vi "WPI_CameraRead MJPG for Dashboard.vi"(6 "Camera Settings":T2={"fps"=30, "compression"=30, "Image Size"=enum."320x240"}, 7 "port":u16=1180, 8 "Rec Mode":u16(ring) items=["O", "*", "Open Playback Panel"], 9 "Camera IP":string, 10 "Camera Mode":u16(ring) items=["Camera Off", "USB Camera SW", "USB Camera HW", "IP Camera"], 11 "Refnum in":T1) -> (2 "Active":bool, 3 "Refnum out":T1, 4 "FPS":dbl, 5 "Bandwidth (Mbps)":dbl)   [LabVIEW 2015]
uses:
  <vilib>/Rock Robotics/WPI/Camera/WPI_CameraSettings Read MJPG.ctl
  <vilib>/Rock Robotics/WPI/Camera/WPI_CameraImageSize.ctl
  <vilib>/vision/Image Controls.llb/IMAQ Image.ctl
  <vilib>/Rock Robotics/WPI/Dashboard/WPI_DashboardLogging Global.vi
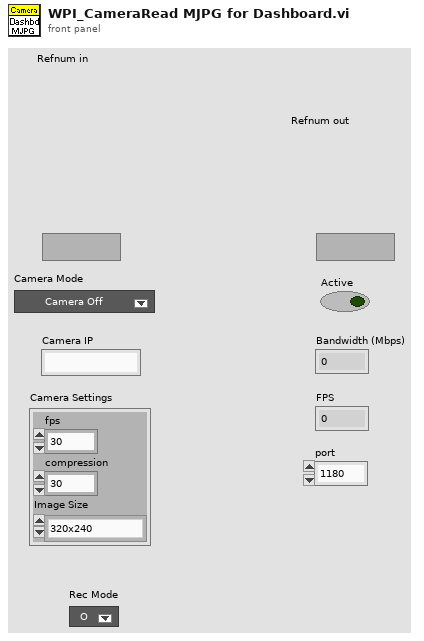
[diagram p1: front panel]
types:
  T1 = typedef "IMAQ Image.ctl" = refnum<image>
  T2 = typedef "WPI_CameraSettings Read MJPG.ctl" = cluster{"fps":i32, "compression":i32, "Image Size":T3}
  T3 = typedef "WPI_CameraImageSize.ctl" = enum16{"640x480", "320x240", "160x120", "Custom"}
  T4 = typedef "IMAQ AVI2 Refnum.ctl" = refnum<k20>
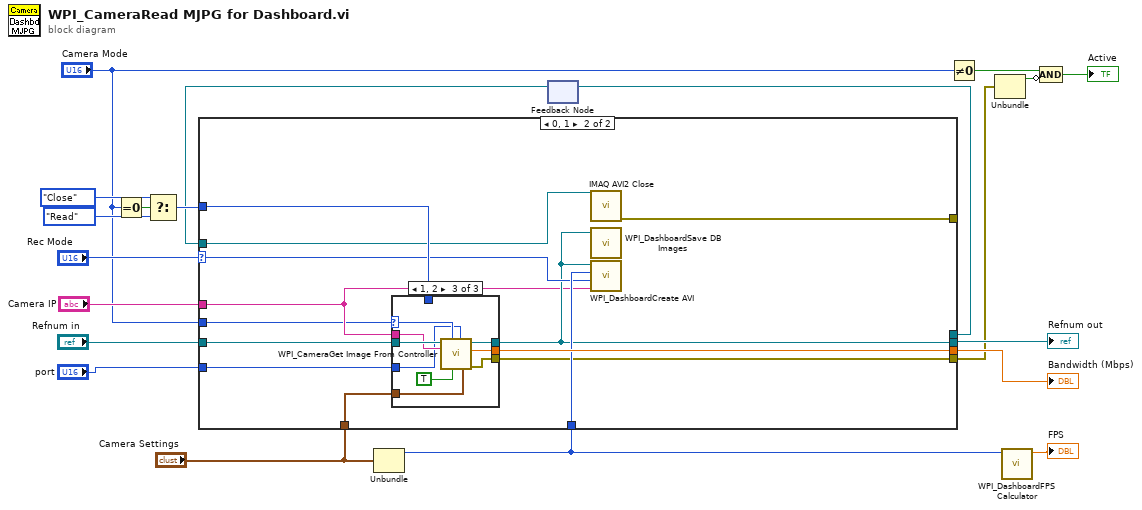
[diagram p0: block diagram]
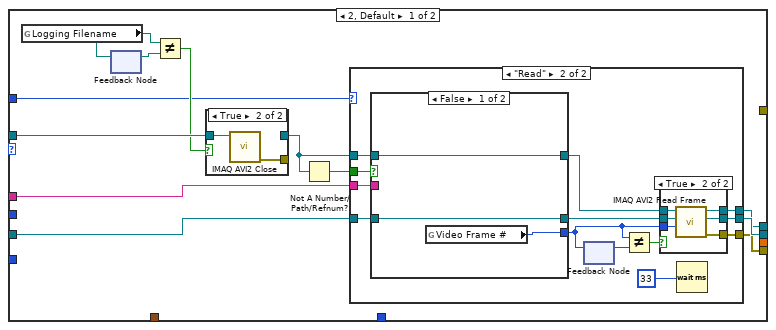
[diagram p2: hidden frame]
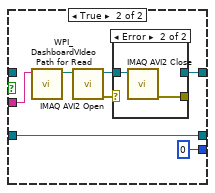
[diagram p5: hidden frame]
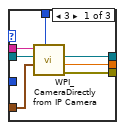
[diagram p8: hidden frame]
diagram:
  n1 = Equal To 0?(x="Camera Mode") -> (x = 0?=w4:bool)
  n2 = Select(t=enum16{"Read", "Reopen", "Close"}."Close" ("Operation"), s=w4, f=enum16{"Read", "Reopen", "Close"}."Read" ("Operation")) -> (s? t:f=w16:enum16{"Read", "Reopen", "Close"})
  n3 = Unbundle("Camera Settings") -> ("fps"=w8:i32)  [unwired: 2 out]
  n4 = feedback #1() -> (w7:T4)  [unwired: 1 in]
  n5 = case shown="0, 1" "Rec Mode" {
    selector: "Rec Mode" -> [_ w79]
    tunnel: "Camera Settings" -> [_ w84]
    tunnel: w16 -> [w21 w83]
    tunnel: [_ w82] -> w13
    tunnel: [w32 w75] -> w9
    tunnel: "Refnum in" -> [w30 w81]
    tunnel: "Camera IP" -> [w27 w74]
    tunnel: w8 -> [_ w80]
    tunnel: w7 -> [w25 w77]
    tunnel: [w29 _] -> w6
    tunnel: [w28 w78] -> w5
    tunnel: [_ w76] -> _
    tunnel: "Camera Mode" -> [_ w73]
    tunnel: "port" -> [_ w72]
    frame 2, Default {
      n6 = global read "WPI_DashboardLogging Global.vi" "Logging Filename"() -> (w24:path)
      n7 = feedback #2() -> (w23:path)  [unwired: 1 in]
      n8 = feedback-in #2(w24) -> ()
      n9 = Not Equal?(x=w24, y=w23) -> (x != y?=w22:bool)
      n10 = case shown="True" w22 {
        tunnel: [w69 _] -> w26
        tunnel: w25 -> [w69 w71]
        tunnel: [_ w70] -> _
        frame False {
        }
        frame True {
          n11 = call "IMAQ AVI2 Close"("AVI Refnum"=w71) -> ("error out"=w70:errorcluster)  [unwired: 10 in]
        }
      }
      n12 = Not A Number/Path/Refnum?(number/path/refnum=w26) -> (NaN/Path/Refnum?=w31:bool)
      n13 = case shown="\"Read\"" w21 {
        tunnel: [w33 w47] -> w32
        tunnel: w31 -> [_ w46]
        tunnel: w30 -> [w33 w43]
        tunnel: [w34 w42] -> w29
        tunnel: [_ w41] -> w28
        tunnel: w27 -> [_ w40]
        tunnel: w26 -> [w34 w39]
        frame "Close", Default {
        }
        frame "Read" {
          n14 = case shown="False" w46 {
            tunnel: [w58 w63] -> w45
            tunnel: w39 -> [w58 _]
            tunnel: [w57 w65] -> w44
            tunnel: w43 -> [w57 w65]
            tunnel: [w56 0 ("Video Frame #")] -> w36
            tunnel: w40 -> [_ w60]
            frame False {
              n15 = global read "WPI_DashboardLogging Global.vi" "Video Frame #"() -> (w56:i32)
            }
            frame True {
              n16 = call <vilib>:"WPI_DashboardVIdeo Path for Read.vi"("Camera IP"=w60) -> ("Video Path"=w59:path)  [unwired: 10 in]
              n17 = call "IMAQ AVI2 Open"("AVI File Path"=w59) -> ("error out"=w64:errorcluster, "AVI Refnum"=w62:T4)  [unwired: 9 in]
              n18 = case shown="Error" w64 {
                tunnel: [w66 _] -> w63
                tunnel: w62 -> [w66 w68]
                tunnel: [_ w67] -> _
                frame No Error {
                }
                frame Error {
                  n19 = call "IMAQ AVI2 Close"("AVI Refnum"=w68) -> ("error out"=w67:errorcluster)  [unwired: 10 in]
                }
              }
            }
          }
          n20 = feedback #3() -> (w37:i32)  [unwired: 1 in]
          n21 = feedback-in #3(w36) -> ()
          n22 = Not Equal?(x=w36, y=w37) -> (x != y?=w38:bool)
          n23 = case shown="True" w38 {
            tunnel: [w48 w55] -> w47
            tunnel: w45 -> [w49 w54]
            tunnel: w44 -> [w48 w53]
            tunnel: [w49 w52] -> w42
            tunnel: [_ w51] -> w41
            tunnel: w36 -> [_ w50]
            frame False {
            }
            frame True {
              n24 = call "IMAQ AVI2 Read Frame"("Frame Number"=w50, "Image"=w53, "AVI Refnum"=w54) -> ("error out"=w51:errorcluster, "Image Out"=w55:T1, "AVI Refnum (duplicate)"=w52:T4)  [unwired: 6 in]
            }
          }
          n25 = Wait (ms)(milliseconds to wait=33) -> ()  [unwired: 1 out]
        }
      }
    }
    frame 0, 1 {
      n26 = case shown="1, 2" w73 {
        selector: w73 -> [_ _ w94]
        tunnel: w84 -> [w91 _ w96]
        tunnel: w83 -> [w85 _ _]
        tunnel: [w89 _ w95] -> w82
        tunnel: w81 -> [w87 w92 w101]
        tunnel: w74 -> [w86 _ w98]
        tunnel: [w90 _ w99] -> w78
        tunnel: [w88 w92 w100] -> w75
        tunnel: w72 -> [_ _ w93]
        frame 3 {
          n27 = call <vilib>:"WPI_CameraDirectly from IP Camera.vi"("Operation"=w85, "Camera Settings"=w91, "Image"=w87, "address"=w86) -> ("error out"=w90:errorcluster, "Bandwidth (Mbps)"=w89:dbl, "Image Out"=w88:T1)  [unwired: 5 in]
        }
        frame Default {
        }
        frame 1, 2 {
          n28 = call "WPI_CameraGet Image From Controller.vi"("Camera Settings"=w96, "port"=w93, "USB"=TRUE, "Camera Mode"=w94, "Controller Address"=w98, "Image"=w101) -> ("error out"=w99:errorcluster, "Bandwidth (Mbps)"=w95:dbl, "Image Out"=w100:T1)  [unwired: 3 in]
        }
      }
      n29 = call "IMAQ AVI2 Close"("AVI Refnum"=w77) -> ("error out"=w76:errorcluster)  [unwired: 10 in]
      n30 = call <vilib>:"WPI_DashboardSave DB Images.vi"("Image"=w75) -> ()  [unwired: 3 in]
      n31 = call <vilib>:"WPI_DashboardCreate AVI.vi"("Camera IP"=w74, "Recording"=w79, "frames per seconds"=w80, "Image"=w75) -> ()  [unwired: 8 in]
    }
  }
  "Bandwidth (Mbps)" <- w13
  "Refnum out" <- w9
  n32 = feedback-in #1(w6) -> ()
  n33 = Not Equal To 0?(x="Camera Mode") -> (x != 0?=w3:bool)
  n34 = Unbundle(w5) -> ("status"=w17:bool)  [unwired: 2 out]
  n35 = call <vilib>:"WPI_DashboardFPS Calculator.vi"("Average Count"=w8) -> ("fps"=→"FPS":dbl)  [unwired: 10 in]
  n36 = Compound Arithmetic op=AND(w3, invert w17) -> (→"Active":bool)
